vi "Table Workspace Tool.vi"() -> ()   [LabVIEW 2012, in "TableSupportLib.lvlib"]
doc: "Sample numeric display item."
uses:
  TableSupportLib.lvlib
  NationalInstruments.VeriStand.SystemStorage
  SubVIs/Table_StateControl.ctl
  SubVIs/Table_ToolConfiguration_Action.ctl
  SubVIs/Table_StateInformation.ctl
  SubVIs/Table_ChannelInfoCluster.ctl
  SubVIs/Table_SortArraySettings.ctl
  SubVIs/Table_ListboxSettings.ctl
  SubVIs/Table_Globals.vi
  <vilib>/NI Veristand/Execution/Workspace/NI VeriStand - Set Single Channel Value.vi
  <vilib>/NI Veristand/Execution/Workspace/NI_VS Workspace ExecutionAPI.lvlib
panel:
  in  "NIVS.Project File Path":path
  in  "NIVS.Workspace Event":refnum<event-registration>
  in  "Value":dbl
  in  "Listbox":i32(listbox)
  in  "NIVS.Gateway IP Address":string
  in  "NIVS.System Definition Root":refnum<k24>
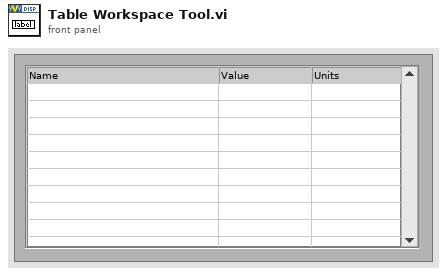
[diagram p1: front panel]
types:
  T1 = typedef "TableSupportLib.lvlib/Table_StateControl.ctl" = enum16{"Init", "Run"}
  T2 = typedef "NI_VS Workspace ExecutionAPI.lvlib/WorkspaceAPI.ctl" = refnum<k24>
  T3 = typedef "NI_VS Workspace ExecutionAPI.lvlib/SystemStateEventRef.ctl" = cluster{"CustDatRef":refnum<user-event>, "EvtRef":refnum<k27>}
  T4 = typedef "NI_VS Workspace ExecutionAPI.lvlib/SystemStateRegEventRef.ctl" = refnum<event-registration>
  T5 = cluster{"NIVS.Workspace Event":refnum<event-registration>, "SystemChangeEventRef":T4}
  T6 = typedef "TableSupportLib.lvlib/Table_ToolConfiguration_Action.ctl" = enum16{"Read", "Write"}
  T7 = typedef "TableSupportLib.lvlib/Table_StateInformation.ctl" = cluster{"Channel Selection":T8[], "Widths":dbl[], "Sort Info":T9, "Listbox Settings":T10}
  T8 = typedef "TableSupportLib.lvlib/Table_ChannelInfoCluster.ctl" = cluster{"NodePath":string, "Name":string, "Units":string, "Enabled":bool}
  T9 = typedef "TableSupportLib.lvlib/Table_SortArraySettings.ctl" = cluster{"Order":enum16{"ascending", "descending"}, "Column":i32}
  T10 = typedef "TableSupportLib.lvlib/Table_ListboxSettings.ctl" = cluster{"Font":u32, "Bold":bool, "Poll Rate":u32, "Enable Limits":bool, "Path":path}
  T11 = typedef "lveventtype.ctl" = enum32{"Null", "Timeout", "Annotation Menu Selection", "Annotation Menu Selection?", "App Instance Close", "App Instance Close?", "Autoscale Range Change", "Cell Edit", "Cell Edit?", "Cursor Grab", "Cursor Grab?", "Cursor Menu Selection", "Cursor Menu Selection?", "Cursor Move", "Cursor Release", "Data Change", "Direction Change", "Display State Change", "Drag Ended", "Drag Enter", "Drag Leave", "Drag Over", "Drag Source Update", "Drag Starting", "Drag Starting?", "Drop", "Exec State Change", "Key Down", "Key Down?", "Key Repeat", "Key Repeat?", "Key Up", "Listbox Double Click", "Menu Activation?", "Menu Selection (App)", "Menu Selection? (App)", "Menu Selection (User)", "Mouse Down", "Mouse Down?", "Mouse Enter", "Mouse Leave", "Mouse Move", "Mouse Up", "NI Security User Change (App)", "Pane Size", "Panel Close", "Panel Close?", "Panel Resize", "Plot Attribute Change", "Scale Range Change", "Shortcut Menu Activation?", "Shortcut Menu Selection (App)", "Shortcut Menu Selection? (App)", "Shortcut Menu Selection (User)", "Tree Double Click", "Tree Drag", "Tree Drag?", "Tree Drop", "Tree Drop?", "Tree Item Close", "Tree Item Close?", "Tree Item Open", "Tree Item Open?", "Value Change"}
  T12 = typedef "LVPoint32TypeDef.ctl" = cluster{"Horizontal":i32, "Vertical":i32}
  T13 = typedef "LVRowAndColumnTypeDef.ctl" = cluster{"Row":i32, "Column":i32}
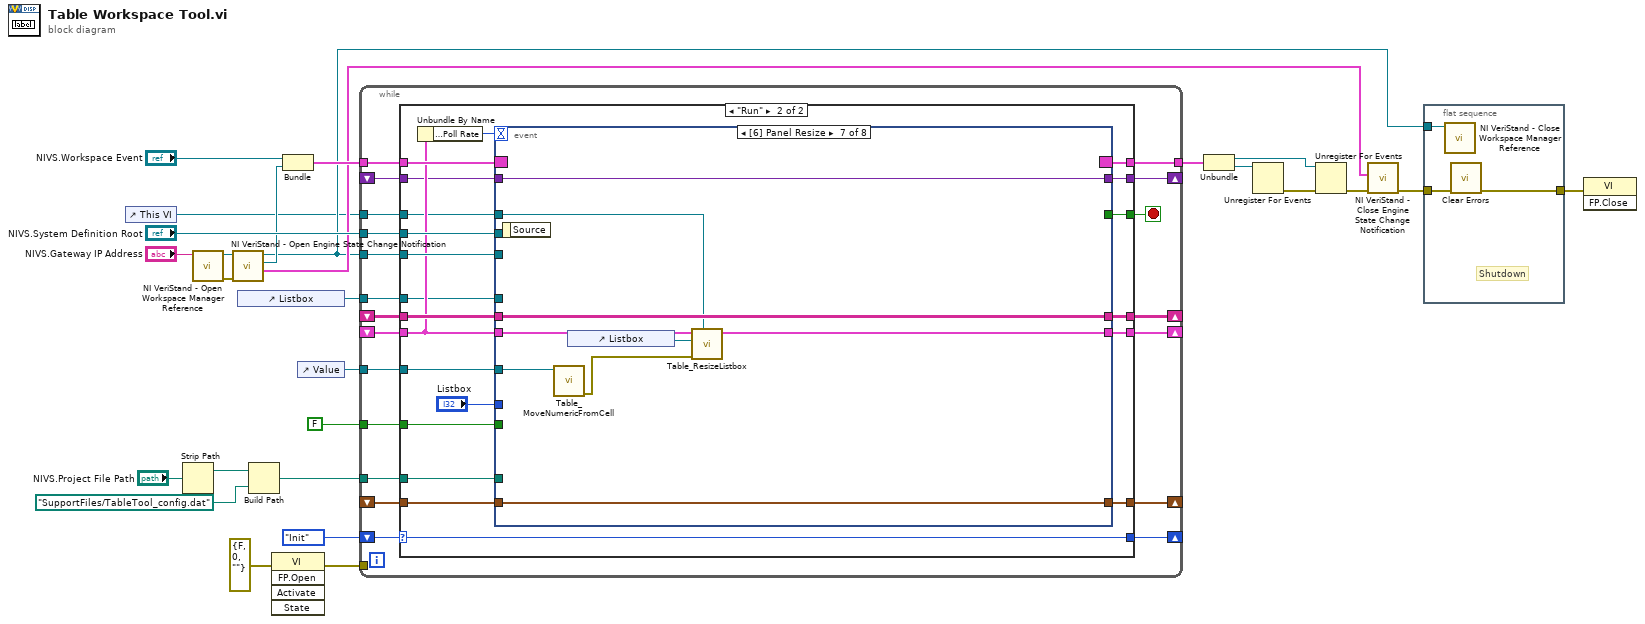
[diagram p0: block diagram]
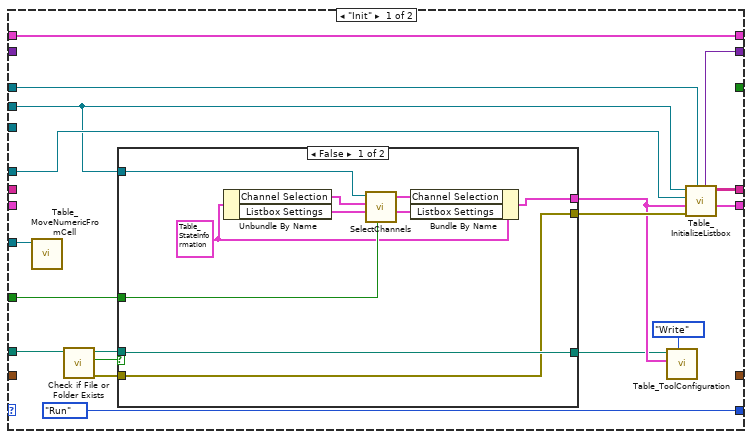
[diagram p2: hidden frame]
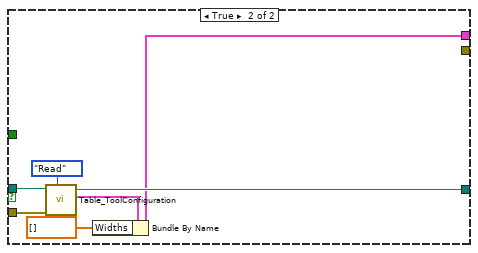
[diagram p3: hidden frame]
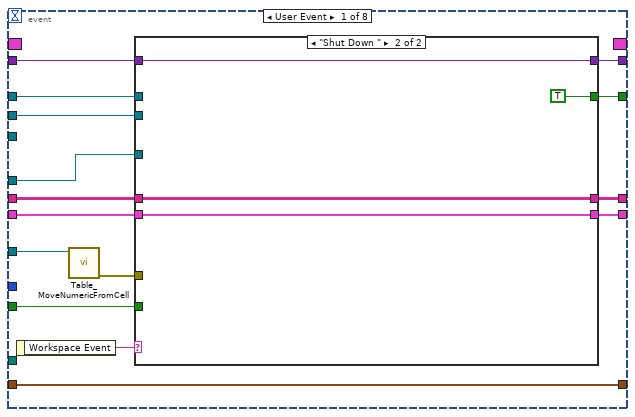
[diagram p4: hidden frame]
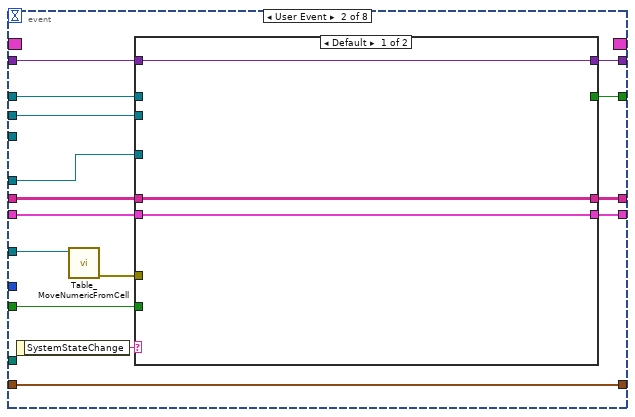
[diagram p6: hidden frame]
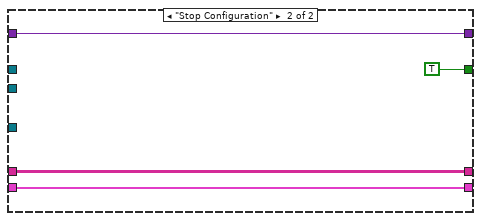
[diagram p7: hidden frame]
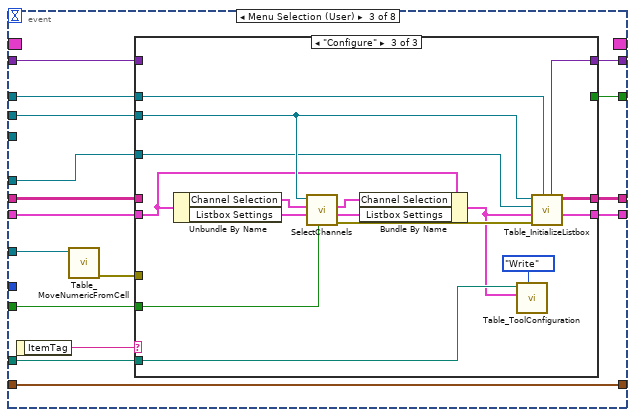
[diagram p8: hidden frame]
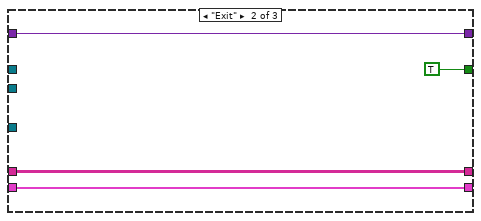
[diagram p10: hidden frame]
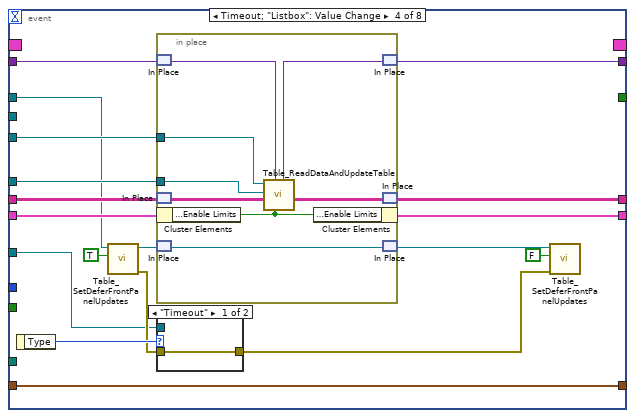
[diagram p11: hidden frame]
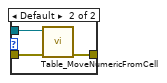
[diagram p12: hidden frame]
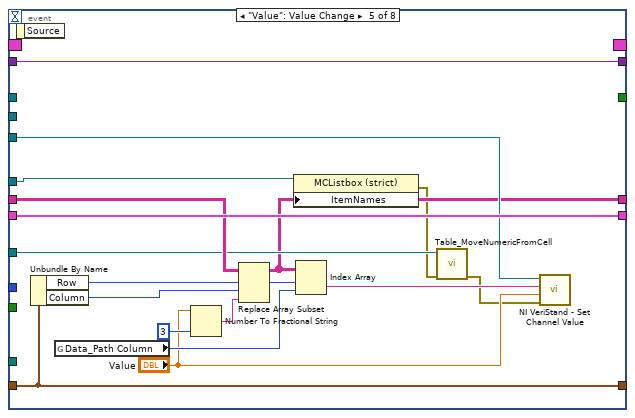
[diagram p13: hidden frame]
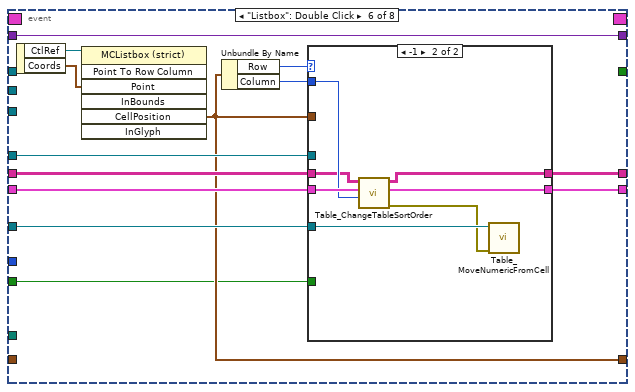
[diagram p14: hidden frame]
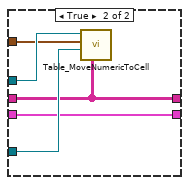
[diagram p16: hidden frame]
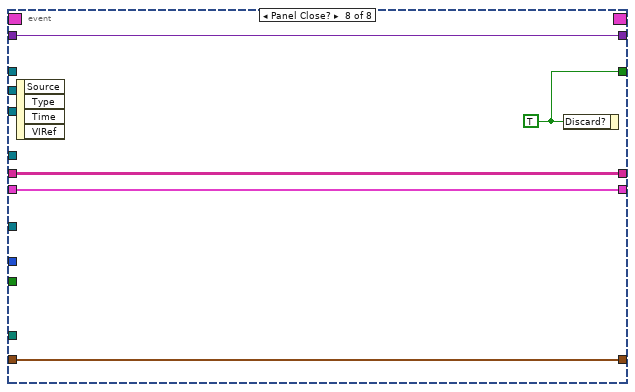
[diagram p17: hidden frame]
diagram:
  n1 = control-ref of="This VI"() -> (w1:refnum<vi>)
  n2 = Strip Path(path="NIVS.Project File Path") -> (stripped path=w4:path)  [unwired: 1 out]
  n3 = call <vilib>:"NI VeriStand - Open Workspace Manager Reference.vi"("Gateway IP Address (\"\": localhost)"="NIVS.Gateway IP Address") -> ("error out"=w7:errorcluster, "WorkspaceManager"=w20:T2)  [unwired: 9 in]
  n4 = call <vilib>:"NI VeriStand - Open Engine State Change Notification.vi"("error in (no error)"=w7, "WorkspaceManager in"=w20) -> ("SystemStateRefs"=w10:T3, "SystemChangeEventRef"=w19:T4, "WorkspaceManager out"=w9:T2)  [unwired: 6 in, 1 out]
  n5 = control-ref of="Listbox"() -> (w24:refnum<vi>)
  n6 = Build Path(base path=w4, name or relative path=path "SupportFiles/TableTool_config.dat" ("stripped path")) -> (appended path=w2:path)
  n7 = invoke class="VI" method="FP.Open"(error in=errorcluster {"status"=FALSE, "code"=0, "source"=""} ("error out")) -> (error out=w6:errorcluster)  [unwired: 4 in, 4 out]
  n8 = Bundle("NIVS.Workspace Event"="NIVS.Workspace Event", "SystemChangeEventRef"=w19) -> (w17:T5)  [unwired: 1 in]
  n9 = control-ref of="Value"() -> (w23:refnum<vi>)
  n10 = while {
    tunnel: w17 -> [w47]
    tunnel: [w45] -> w16
    tunnel: "NIVS.System Definition Root" -> [w44]
    shift-right: [w41] -> _
    shift-left: _ -> [w43]
    tunnel: w9 -> [w42]
    shift-right: [w40] -> _
    shift-left: _ -> [w39]
    shift-right: [w37] -> _
    shift-left: Table_StateControl."Init" -> [w38]
    shift-right: [w36] -> _
    shift-left: _ -> [w35]
    tunnel: w1 -> [w34]
    tunnel: w24 -> [w33]
    tunnel: w23 -> [w32]
    shift-right: [w31] -> _
    shift-left: _ -> [w30]
    tunnel: FALSE ("Controls Only?") -> [w29]
    tunnel: w6 -> [_]
    tunnel: w2 -> [w28]
    stop <- w46 stop-if-true
    n11 = case shown="\"Run\"" w38 {
      selector: w38 -> [_ w95]
      tunnel: w47 -> [w65 w103]
      tunnel: [_ w102] -> w46
      tunnel: [w65 w101] -> w45
      tunnel: w44 -> [w56 w100]
      tunnel: w43 -> [_ w94]
      tunnel: w42 -> [_ w99]
      tunnel: [w63 w98] -> w41
      tunnel: [w62 w97] -> w40
      tunnel: w39 -> [_ w96]
      tunnel: [Table_StateControl."Run" w95] -> w37
      tunnel: [w61 w92] -> w36
      tunnel: w35 -> [_ w91]
      tunnel: w34 -> [w60 w90]
      tunnel: w33 -> [w59 w88]
      tunnel: w32 -> [w58 w87]
      tunnel: [_ w86] -> w31
      tunnel: w30 -> [_ w85]
      tunnel: w29 -> [w57 w84]
      tunnel: w28 -> [w54 w83]
      frame "Init" {
        n12 = call "Table_MoveNumericFromCell.vi"("Digital in"=w58) -> ()  [unwired: 10 in, 1 out]
        n13 = call <vilib>:"Check if File or Folder Exists.vi"("path"=w54) -> ("error out"=w49:errorcluster, "file or folder exists?"=w48:bool, "dup path"=w53:path)  [unwired: 8 in]
        n14 = case shown="False" w48 {
          tunnel: w57 -> [w69 _]
          tunnel: w56 -> [w68 _]
          tunnel: [w74 _] -> w55
          tunnel: w53 -> [w75 w82]
          tunnel: [w67 w76] -> w51
          tunnel: [w75 w81] -> w50
          tunnel: w49 -> [w74 w80]
          frame False {
            w66 = T7 {"Channel Selection"=[], "Widths"=[], "Sort Info"={"Order"=enum."ascending", "Column"=0}, "Listbox Settings"={"Font"=13, "Bold"=FALSE, "Poll Rate"=200, "Enable Limits"=FALSE, "Path"=path ""}}
            n15 = Unbundle By Name(w66) -> ("Channel Selection"=w73:T8[], "Listbox Settings"=w70:T10)
            n16 = call "SelectChannels.vi"("Controls Only?"=w69, "Listbox Settings"=w70, "Previous Selection"=w73, "Root.BaseNodeType"=w68) -> ("Listbox Settings Out"=w71:T10, "Channel Selection"=w72:T8[])  [unwired: 5 in, 1 out]
            n17 = Bundle By Name(cluster=w66, "Channel Selection"=w72, "Listbox Settings"=w71) -> (w67:T7)
          }
          frame True {
            n18 = call "Table_ToolConfiguration.vi"("Action"=Table_ToolConfiguration_Action."Read", "error in"=w80, "datalog path (use dialog)"=w82) -> ("Custom Data Out"=w77:T7, "path out"=w81:path)  [unwired: 6 in, 1 out]
            n19 = Bundle By Name(cluster=w77, "Widths"=dbl[] []) -> (w76:T7)
          }
        }
        n20 = call "Table_ToolConfiguration.vi"("Action"=Table_ToolConfiguration_Action."Write", "Custom Data"=w51, "datalog path (use dialog)"=w50) -> ()  [unwired: 6 in, 3 out]
        n21 = call "Table_InitializeListbox.vi"("This VI"=w60, "error in (no error)"=w55, "State Information"=w51, "Listbox Ref"=w59, "NIVS.System Definition Root"=w56) -> ("State Information Out"=w63:T7, "Sorted Array out"=w62:string[][], "Limit Settings"=w61:variant)  [unwired: 2 in, 2 out]
      }
      frame "Run" {
        n22 = Unbundle By Name(w94) -> ("Listbox Settings.Poll Rate"=w93:u32)
        n23 = event shown="[6] Panel Resize" {
          selector: w103 -> [_ _ _ _ _ _ _ _]
          dyn-events: [_ _ _ _ _ _ _ _] -> w101
          timeout: w93 -> [_ _ _ _ _ _ _ _]
          tunnel: [w118 w140 w163 _ _ _ _ w278] -> w102
          tunnel: w100 -> [w117 w139 w162 _ _ _ _ _]
          tunnel: w94 -> [w116 w138 w161 w203 w232 w243 w274 w282]
          tunnel: w99 -> [_ _ _ w204 w226 _ _ _]
          tunnel: [w115 w137 w160 w202 w232 w242 w275 w282] -> w98
          tunnel: [w114 w136 w159 w198 w219 w240 w277 w281] -> w97
          tunnel: w96 -> [w113 w135 w158 w199 w225 w241 w277 w281]
          tunnel: [w112 w134 w157 w200 w233 w239 w273 w280] -> w92
          tunnel: w91 -> [w111 w133 w156 w201 w233 w239 w273 w280]
          tunnel: w90 -> [w110 w132 w155 w195 _ _ w272 _]
          tunnel: "Listbox" -> [_ _ _ _ _ _ _ _]
          tunnel: w88 -> [w109 w131 w154 w197 w220 w238 _ _]
          tunnel: w87 -> [w107 w129 w152 w187 w221 w237 w270 _]
          tunnel: [w108 w130 w153 w191 w231 w236 w271 w279] -> w86
          tunnel: w85 -> [w108 w130 w153 w191 w231 _ w271 w279]
          tunnel: w84 -> [w105 w127 w150 _ _ w234 _ _]
          tunnel: w83 -> [_ _ w148 _ _ _ _ _]
          event User Event {
            n24 = event-data() -> ("Workspace Event"=w104:string)  [unwired: 1 out]
            n25 = call "Table_MoveNumericFromCell.vi"("Digital in"=w107) -> ("error out"=w106:errorcluster)  [unwired: 10 in]
            n26 = case shown="\"Shut Down \"" w104 {
              tunnel: [_ TRUE] -> w118
              tunnel: w117 -> [_ _]
              tunnel: w116 -> [w121 w124]
              tunnel: [w121 w124] -> w115
              tunnel: [w120 w123] -> w114
              tunnel: w113 -> [w120 w123]
              tunnel: [w119 w122] -> w112
              tunnel: w111 -> [w119 w122]
              tunnel: w110 -> [_ _]
              tunnel: w109 -> [_ _]
              tunnel: w106 -> [_ _]
              tunnel: w105 -> [_ _]
              frame Default {
              }
              frame "Shut Down " {
              }
            }
          }
          event User Event {
            n27 = event-data() -> ("SystemStateChange"=w126:string)  [unwired: 1 out]
            n28 = call "Table_MoveNumericFromCell.vi"("Digital in"=w129) -> ("error out"=w128:errorcluster)  [unwired: 10 in]
            n29 = case shown="Default" w126 {
              tunnel: [_ TRUE] -> w140
              tunnel: w139 -> [_ _]
              tunnel: w138 -> [w143 w146]
              tunnel: [w143 w146] -> w137
              tunnel: [w142 w145] -> w136
              tunnel: w135 -> [w142 w145]
              tunnel: [w141 w144] -> w134
              tunnel: w133 -> [w141 w144]
              tunnel: w132 -> [_ _]
              tunnel: w131 -> [_ _]
              tunnel: w128 -> [_ _]
              tunnel: w127 -> [_ _]
              frame Default {
              }
              frame "Stop Configuration" {
              }
            }
          }
          event Menu Selection (User) {
            n30 = event-data() -> ("ItemTag"=w149:string)  [unwired: 1 out]
            n31 = call "Table_MoveNumericFromCell.vi"("Digital in"=w152) -> ("error out"=w151:errorcluster)  [unwired: 10 in]
            n32 = case shown="\"Configure\"" w149 {
              tunnel: [_ TRUE _] -> w163
              tunnel: w162 -> [_ _ w185]
              tunnel: w161 -> [w166 w169 w183]
              tunnel: [w166 w169 w180] -> w160
              tunnel: [w165 w168 w181] -> w159
              tunnel: w158 -> [w165 w168 _]
              tunnel: [w164 w167 w177] -> w157
              tunnel: w156 -> [w164 w167 _]
              tunnel: w155 -> [_ _ w176]
              tunnel: w154 -> [_ _ w175]
              tunnel: w151 -> [_ _ _]
              tunnel: w150 -> [_ _ w174]
              tunnel: w148 -> [_ _ w172]
              frame Default {
              }
              frame "Exit" {
              }
              frame "Configure" {
                n33 = Unbundle By Name(w183) -> ("Channel Selection"=w186:T8[], "Listbox Settings"=w178:T10)
                n34 = call "SelectChannels.vi"("Controls Only?"=w174, "Listbox Settings"=w178, "Previous Selection"=w186, "Root.BaseNodeType"=w185) -> ("error out"=w184:errorcluster, "Listbox Settings Out"=w179:T10, "Channel Selection"=w182:T8[])  [unwired: 5 in]
                n35 = Bundle By Name(cluster=w183, "Channel Selection"=w182, "Listbox Settings"=w179) -> (w171:T7)
                n36 = call "Table_ToolConfiguration.vi"("Action"=Table_ToolConfiguration_Action."Write", "Custom Data"=w171, "datalog path (use dialog)"=w172) -> ()  [unwired: 6 in, 3 out]
                n37 = call "Table_InitializeListbox.vi"("This VI"=w176, "error in (no error)"=w184, "State Information"=w171, "Listbox Ref"=w175, "NIVS.System Definition Root"=w185) -> ("State Information Out"=w180:T7, "Sorted Array out"=w181:string[][], "Limit Settings"=w177:variant)  [unwired: 2 in, 2 out]
              }
            }
          }
          event Timeout; "Listbox": Value Change {
            n38 = event-data() -> ("Type"=w189:T11)  [unwired: 1 out]
            n39 = call "Table_SetDeferFrontPanelUpdates.vi"("Defer Panel Updates"=TRUE, "VI Ref"=w195) -> ("error out"=w188:errorcluster, "VI Ref out"=w194:refnum<vi>)  [unwired: 8 in]
            n40 = in-place {
              in-place-border: w204 -> [w216]
              in-place-border: w197 -> [w210]
              n41 = in-place-match #1(w201) -> (w214:variant)
              n42 = in-place-match #2(w199) -> (w212:string[][])
              n43 = in-place-cluster #3(w203) -> ("Listbox Settings.Enable Limits"=w215:bool)
              n44 = in-place-match #4(w194) -> (w209:refnum<vi>)
              n45 = call "Table_ReadDataAndUpdateTable.vi"("Enable Limits"=w215, "Limit Settings"=w214, "Data"=w212, "Listbox Ref"=w210, "WorkspaceManager"=w216) -> ("Data Out"=w211:string[][], "Limit Settings Out"=w213:variant)  [unwired: 3 in, 2 out]
              n46 = in-place-cluster #3("Listbox Settings.Enable Limits"=w215) -> (w202:T7)
              n47 = in-place-match #1(w213) -> (w200:variant)
              n48 = in-place-match #2(w211) -> (w198:string[][])
              n49 = in-place-match #4(w209) -> (w193:refnum<vi>)
            }
            n50 = case shown="\"Timeout\"" w189 {
              tunnel: [w205 w208] -> w190
              tunnel: w188 -> [w205 w207]
              tunnel: w187 -> [_ w206]
              frame "Timeout" {
              }
              frame Default {
                n51 = call "Table_MoveNumericFromCell.vi"("error in (no error)"=w207, "Digital in"=w206) -> ("error out"=w208:errorcluster)  [unwired: 9 in]
              }
            }
            n52 = call "Table_SetDeferFrontPanelUpdates.vi"("error in (no error)"=w190, "Defer Panel Updates"=FALSE, "VI Ref"=w193) -> ()  [unwired: 7 in, 2 out]
          }
          event "Value": Value Change {
            n53 = event-data() -> ()  [unwired: 2 out]
            n54 = Unbundle By Name(w231) -> ("Row"=w229:i32, "Column"=w230:i32)
            n55 = global read "Table_Globals.vi" "Data_Path Column"() -> (w228:i32)
            n56 = Number To Fractional String(number="Value", precision (6)=i16 3) -> (F-format string=w222:string)  [unwired: 2 in]
            n57 = Replace Array Subset(array=w225, new element=w222, index (row)=w229, index (col)=w230) -> (w219:string[][])
            n58 = property on="Property Node" class="MCListbox (strict)"(reference=w220, "ItemNames"=w219) -> (error out=w218:errorcluster)  [unwired: 1 in, 1 out]
            n59 = Index Array(array=w219, index (row)=w229, index (col)=w228) -> (element=w227:string)
            n60 = call "Table_MoveNumericFromCell.vi"("error in (no error)"=w218, "Digital in"=w221) -> ("error out"=w217:errorcluster)  [unwired: 9 in]
            n61 = call-poly <vilib>:"NI VeriStand - Set Channel Value.vi"("error in (no error)"=w217, "Value"="Value", "Channel"=w227, "WorkspaceManager in"=w226) -> ()  [unwired: 6 in, 2 out]
          }
          event "Listbox": Double Click {
            n62 = event-data() -> ("CtlRef"=w246:refnum<vi>, "Coords"=w245:T12)  [unwired: 1 out]
            n63 = invoke class="MCListbox (strict)" method="Point To Row Column"(reference=w246, "Point"=w245) -> ("CellPosition"=w236:T13)  [unwired: 5 in, 6 out]
            n64 = Unbundle By Name(w236) -> ("Row"=w235:i32, "Column"=w244:i32)
            n65 = case shown="-1" w235 {
              tunnel: w244 -> [_ w265]
              tunnel: w243 -> [w247 w268]
              tunnel: [w248 w267] -> w242
              tunnel: w241 -> [w253 w264]
              tunnel: [w249 w266] -> w240
              tunnel: w238 -> [w254 _]
              tunnel: w236 -> [w252 _]
              tunnel: w237 -> [w251 w263]
              tunnel: w234 -> [w250 _]
              frame Default {
                n66 = case shown="False" w250 {
                  tunnel: w254 -> [_ w261]
                  tunnel: w253 -> [w256 w258]
                  tunnel: w252 -> [_ w260]
                  tunnel: w251 -> [_ w259]
                  tunnel: [w256 w258] -> w249
                  tunnel: [w255 w257] -> w248
                  tunnel: w247 -> [w255 w257]
                  frame False {
                  }
                  frame True {
                    n67 = call "Table_MoveNumericToCell.vi"("Data"=w258, "Numeric"=w259, "Cell Position"=w260, "Listbox"=w261) -> ()  [unwired: 7 in, 1 out]
                  }
                }
              }
              frame -1 {
                n68 = call "Table_ChangeTableSortOrder.vi"("Column"=w265, "State Information in"=w268, "Data In"=w264) -> ("error out"=w262:errorcluster, "State Information out"=w267:T7, "Data Out"=w266:string[][])  [unwired: 6 in]
                n69 = call "Table_MoveNumericFromCell.vi"("error in (no error)"=w262, "Digital in"=w263) -> ()  [unwired: 9 in, 1 out]
              }
            }
          }
          event Panel Resize {
            n70 = event-data() -> ()  [unwired: 2 out]
            n71 = call "Table_MoveNumericFromCell.vi"("Digital in"=w270) -> ("error out"=w269:errorcluster)  [unwired: 10 in]
            n72 = control-ref of="Listbox"() -> (w276:refnum<vi>)
            n73 = call "Table_ResizeListbox.vi"("VI in"=w272, "error in (no error)"=w269, "Listbox Ref"=w276, "State Information"=w274) -> ("State Information Out"=w275:T7)  [unwired: 5 in, 2 out]
          }
          event Panel Close? {
            w278 = TRUE ("Discard?")
            n74 = event-data() -> ()  [unwired: 5 out]
            n75 = event-data("Discard?"=w278) -> ()  [unwired: 1 in, 1 out]
          }
        }
      }
    }
  }
  n76 = Unbundle(w16) -> ("NIVS.Workspace Event"=w15:refnum<event-registration>, "SystemChangeEventRef"=w13:T4)
  n77 = Unregister For Events(event registration refnum=w13) -> (error out=w14:errorcluster)  [unwired: 1 in]
  n78 = Unregister For Events(event registration refnum=w15, error in=w14) -> (error out=w12:errorcluster)
  n79 = call <vilib>:"NI VeriStand - Close Engine State Change Notification.vi"("error in (no error)"=w12, "SystemStateRefs"=w10) -> ("error out"=w11:errorcluster)  [unwired: 9 in]
  n80 = flat-sequence {
    tunnel: w11 -> [w284]
    tunnel: w9 -> [w285]
    tunnel: [w283] -> w8
    frame #0 {
      # "Shutdown"
      n81 = call <vilib>:"NI VeriStand - Close Workspace Manager Reference.vi"("WorkspaceManager"=w285) -> ()  [unwired: 10 in, 1 out]
      n82 = call <vilib>:"Clear Errors.vi"("error in (no error)"=w284) -> ("error out"=w283:errorcluster)  [unwired: 6 in]
    }
  }
  n83 = invoke class="VI" method="FP.Close"(error in=w8) -> ()  [unwired: 2 in, 3 out]
